vi "Read Exception Status.vi"(8 "error in (no error)":errorcluster, 11 "device data model in":refnum<class "Standard Data Model.lvclass">) -> (0 "error out":errorcluster, 2 "exception status":u8, 3 "device data model out":refnum<class "Standard Data Model.lvclass">)   [LabVIEW 2018, in "SubVIs.lvlib" / "Standard Data Model.lvclass"]
doc: "Reads any exception status set in the device model. The exeption status is a single 8-bit integer."
uses:
  Standard Data Model.lvclass
  Standard Data Model.lvclass/Standard Data Model.ctl
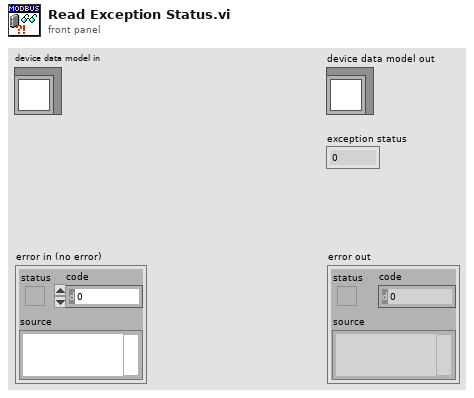
[diagram p1: front panel]
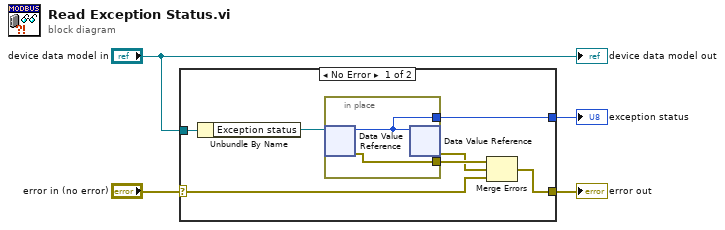
[diagram p0: block diagram]
diagram:
  n1 = case shown="No Error" "error in (no error)" {
    selector: "error in (no error)" -> [w6 w14]
    tunnel: "device data model in" -> [w11 _]
    tunnel: [w10 w14] -> w3
    tunnel: [w8 _] -> w2
    frame No Error {
      n2 = Unbundle By Name(w11) -> ("Exception status"=w9:refnum<data-value>)
      n3 = in-place {
        in-place-border: [w13] -> w8
        in-place-border: [w12] -> w7
        n4 = in-place-dvr #1(w9) -> (w13:u8, w12:errorcluster)
        n5 = in-place-dvr #1(w13) -> (w5:errorcluster)  [unwired: 1 out]
      }
      n6 = Merge Errors(w7, w5, w6) -> (w10:errorcluster)
    }
    frame Error {
    }
  }
  "error out" <- w3
  "exception status" <- w2
  "device data model out" <- "device data model in"
